vi "Construct.vi"(8 "error in (no error)":errorcluster, 11 "CDependencyInspector in":refnum<class "CDependencyInspection.lvclass">) -> (0 "error out":errorcluster, 3 "CDependencyInspector out":refnum<class "CDependencyInspection.lvclass">)   [LabVIEW 2020, in "DependencyInspection.lvlib" / "CDependencyInspection.lvclass"]
uses:
  CDependencyInspection.lvclass
  CDependencyList/CDependencyList.lvclass
  CRuleList/CRuleList.lvclass
  CReporter/CReporter.lvclass
  obj/Addons/ErrorManager.lvlibp/ErrorManager/ErrorManager.lvclass
  CDependencyInspection.lvclass/CDependencyInspection.ctl
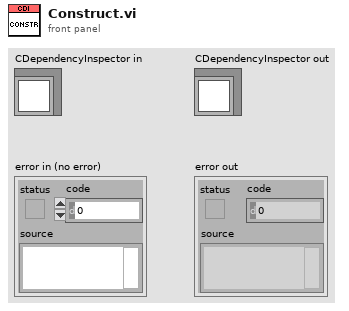
[diagram p1: front panel]
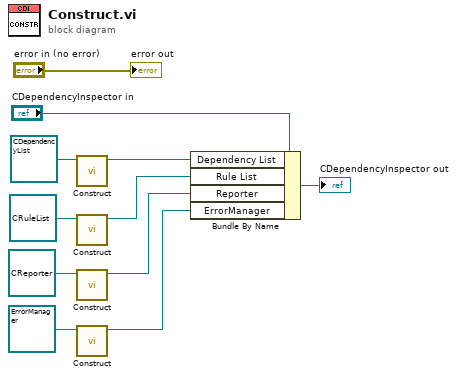
[diagram p0: block diagram]
diagram:
  n1 = call-dynamic "Construct.vi"("CDependencyList in"=refnum<class "CDependencyList.lvclass"> refnum ("Dependency List")) -> ("CDependencyList out"=w7:refnum<class "CDependencyList.lvclass">)  [unwired: 9 in, 1 out]
  n2 = call-dynamic "Construct.vi"("CRuleList in"=refnum<class "CRuleList.lvclass"> refnum ("Rule List")) -> ("CRuleList out"=w5:refnum<class "CRuleList.lvclass">)  [unwired: 9 in, 1 out]
  n3 = call-dynamic "Construct.vi"("CReporter in"=refnum<class "CReporter.lvclass"> refnum ("DGML_Generator_Helper.lvlib:CReporter.lvclass")) -> ("CReporter out"=w3:refnum<class "CReporter.lvclass">)  [unwired: 9 in, 1 out]
  n4 = call-dynamic "Construct.vi"("ErrorManager in"=refnum<class "ErrorManager.lvclass"> refnum) -> ("ErrorManager out"=w1:refnum<class "ErrorManager.lvclass">)  [unwired: 9 in, 1 out]
  n5 = Bundle By Name(cluster="CDependencyInspector in", "Dependency List"=w7, "Rule List"=w5, "Reporter"=w3, "ErrorManager"=w1) -> (→"CDependencyInspector out":refnum<class "CDependencyInspection.lvclass">)
  "error out" <- "error in (no error)"
